vi "External Interface - Get Max & Min.vi"(0 "Ctl Refnum In":refnum<vi>, 1 "VI Refnum In":refnum<vi>, 5 "VI Name":path, 7 "String Control Value":string, 9 "Variant Control Value":variant, 11 "error in":errorcluster, 12 "Control Name":string) -> (3 "VI Refnum Out":refnum<vi>, 4 "Ctl Refnum Out":refnum<vi>, 8 "Message":string, 15 "error out":errorcluster)   [LabVIEW 2010]
panel:
  out "Type":u8
  out "Class Name":string
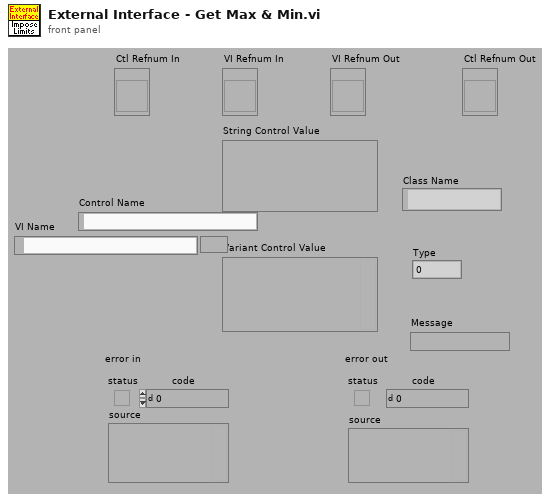
[diagram p1: front panel]
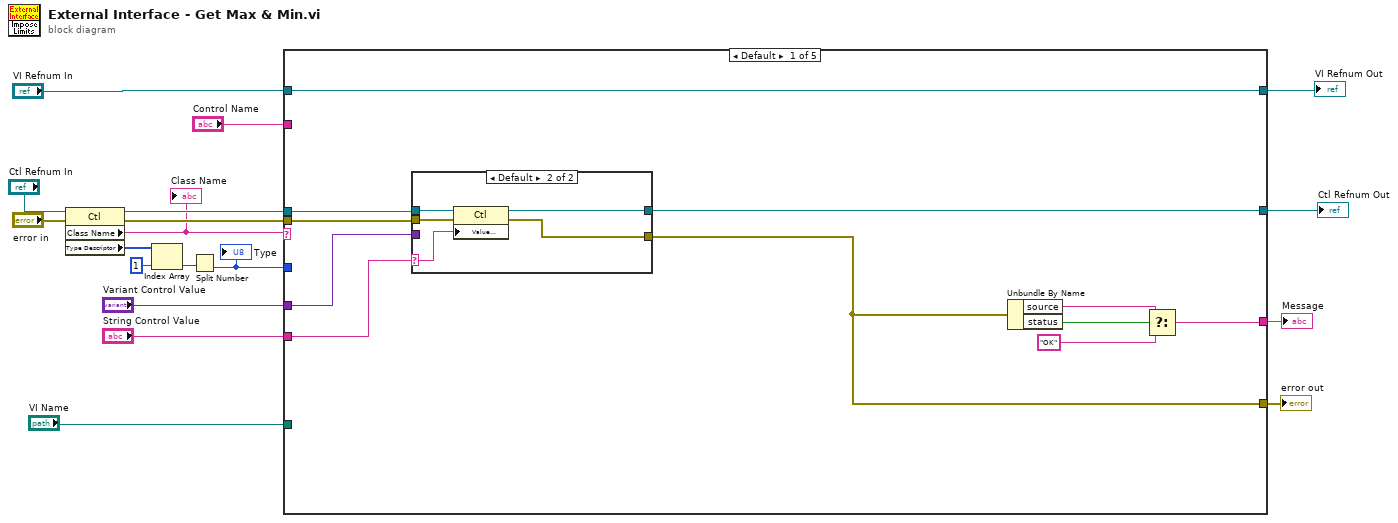
[diagram p0: block diagram]
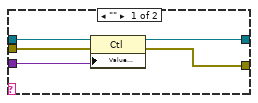
[diagram p2: hidden frame]
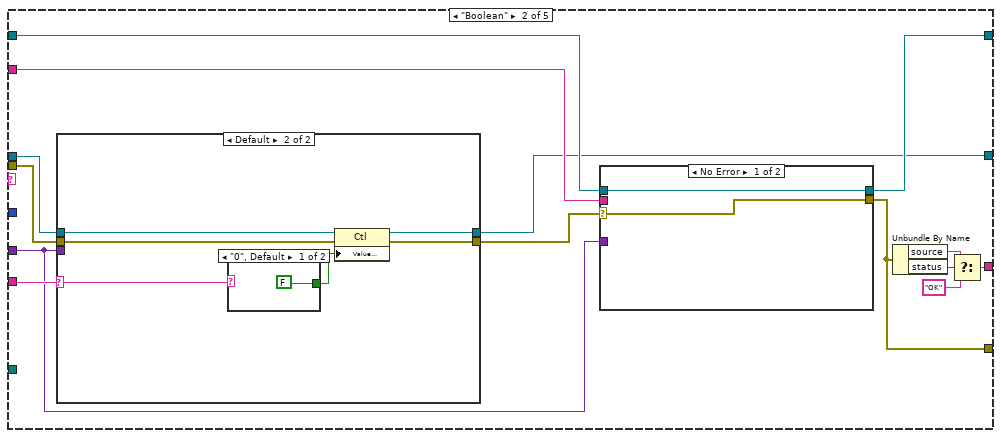
[diagram p3: hidden frame]
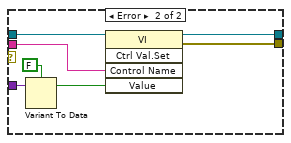
[diagram p4: hidden frame]
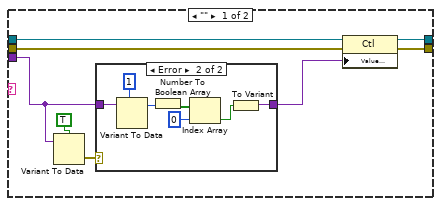
[diagram p5: hidden frame]
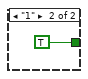
[diagram p7: hidden frame]
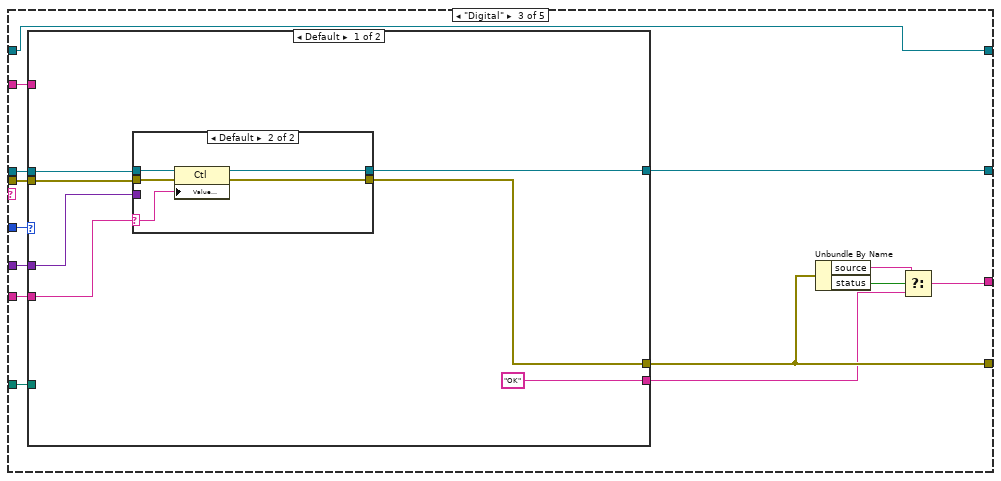
[diagram p8: hidden frame]
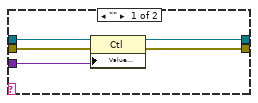
[diagram p9: hidden frame]
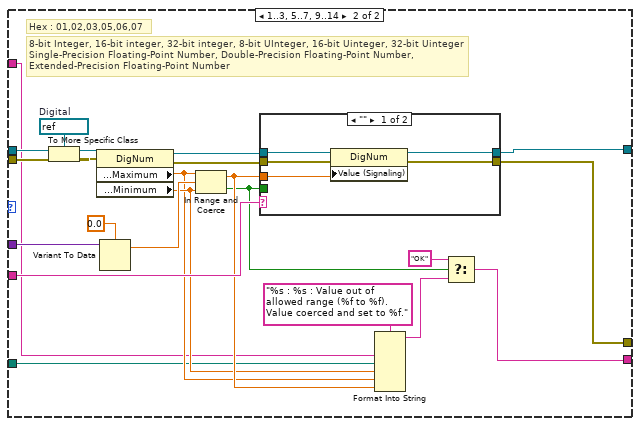
[diagram p10: hidden frame]
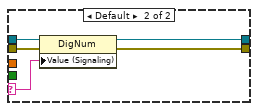
[diagram p11: hidden frame]
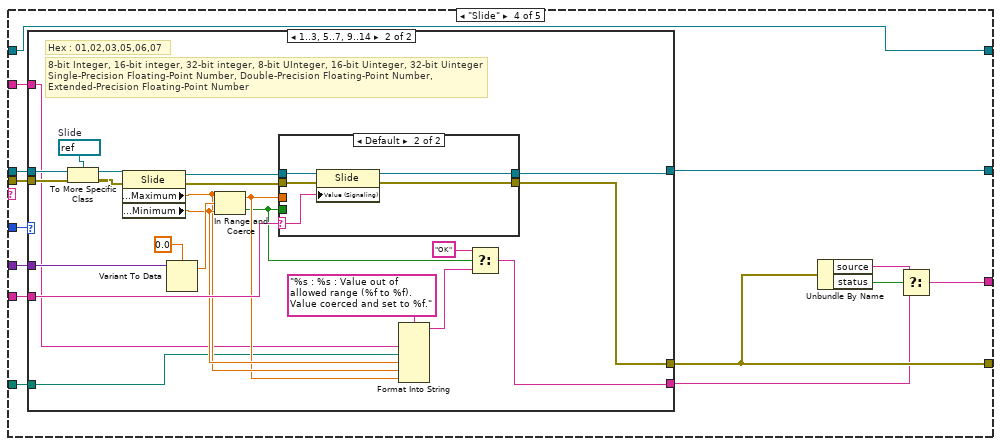
[diagram p12: hidden frame]
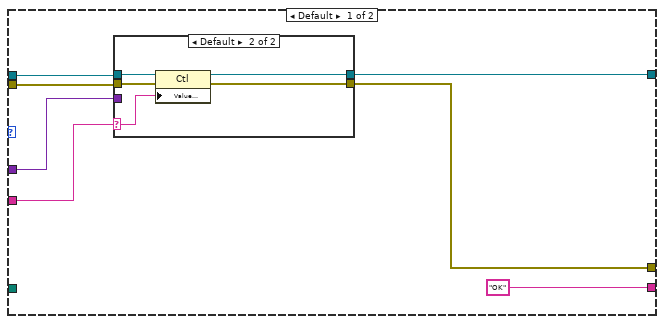
[diagram p13: hidden frame]
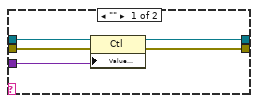
[diagram p14: hidden frame]
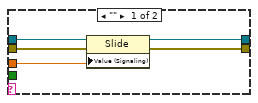
[diagram p15: hidden frame]
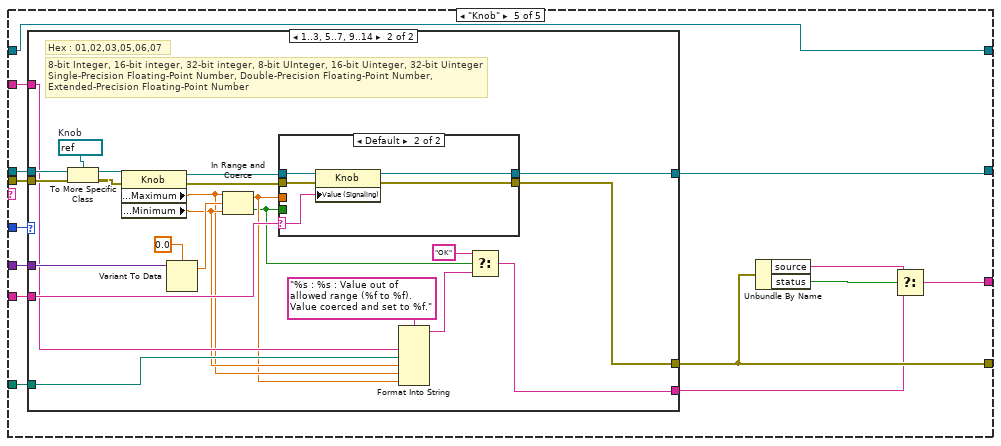
[diagram p16: hidden frame]
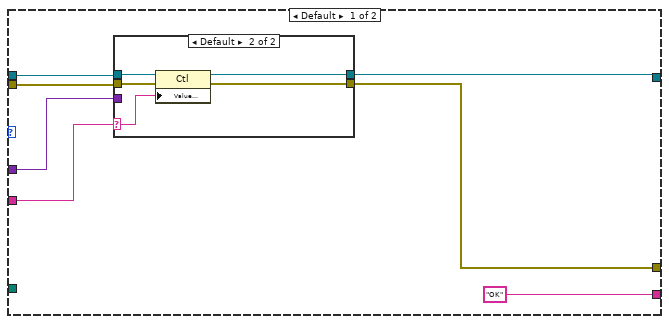
[diagram p17: hidden frame]
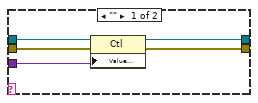
[diagram p18: hidden frame]
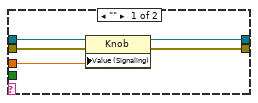
[diagram p19: hidden frame]
diagram:
  n1 = property class="Ctl"(reference="Ctl Refnum In", error in="error in") -> (reference out=w12:refnum<vi>, error out=w11:errorcluster, "Class Name"=w7:string, "Type Descriptor"=w8:i16[])
  "Class Name" <- w7
  n2 = Index Array(array=w8, index=1) -> (element=w17:i16)
  n3 = Split Number(x=w17) -> (lo(x)=w16:u8)  [unwired: 1 out]
  "Type" <- w16
  n4 = case shown="Default" w7 {
    tunnel: w16 -> [_ _ w100 w164 w228]
    tunnel: "Variant Control Value" -> [w27 w49 w99 w163 w227]
    tunnel: "String Control Value" -> [w26 w53 w98 w162 w226]
    tunnel: w12 -> [w29 w52 w97 w161 w225]
    tunnel: w11 -> [w28 w51 w96 w160 w224]
    tunnel: [w19 w44 w92 w157 w220] -> w10
    tunnel: "VI Refnum In" -> [w21 w50 w88 w152 w216]
    tunnel: "Control Name" -> [_ w48 w90 w153 w218]
    tunnel: [w24 w43 w93 w156 w221] -> w4
    tunnel: "VI Name" -> [_ _ w89 w154 w217]
    tunnel: [w21 w42 w88 w152 w216] -> w2
    tunnel: [w20 w40 w87 w151 w215] -> w1
    frame Default {
      n5 = case shown="Default" w26 {
        selector: w26 -> [_ w37]
        tunnel: w29 -> [w34 w39]
        tunnel: w28 -> [w33 w38]
        tunnel: [w31 w36] -> w19
        tunnel: w27 -> [w32 _]
        tunnel: [w30 w35] -> w20
        frame "" {
          n6 = property class="Ctl"(reference=w34, error in=w33, "Value (Signaling)"=w32) -> (reference out=w30:refnum<vi>, error out=w31:errorcluster)
        }
        frame Default {
          n7 = property class="Ctl"(reference=w39, error in=w38, "Value (Signaling)"=w37) -> (reference out=w35:refnum<vi>, error out=w36:errorcluster)
        }
      }
      n8 = Unbundle By Name(w19) -> ("source"=w22:string, "status"=w25:bool)
      n9 = Select(t=w22, s=w25, f="OK") -> (s? t:f=w24:string)
    }
    frame "Boolean" {
      n10 = case shown="Default" w53 {
        selector: w53 -> [_ w82]
        tunnel: w52 -> [w70 w84]
        tunnel: w51 -> [w69 w83]
        tunnel: [w64 w80] -> w41
        tunnel: w49 -> [w65 _]
        tunnel: [w63 w79] -> w40
        frame "" {
          n11 = Variant To Data(Variant=w65, type=TRUE) -> (error out=w68:errorcluster)  [unwired: 1 in, 1 out]
          n12 = case shown="Error" w68 {
            tunnel: w65 -> [w71 w77]
            tunnel: [w71 w73] -> w66
            frame No Error {
            }
            frame Error {
              n13 = Variant To Data(Variant=w77, type=1) -> (data=w76:i32)  [unwired: 1 in, 1 out]
              n14 = Number To Boolean Array(number=w76) -> (Boolean array=w75:bool[])
              n15 = Index Array(array=w75, index=0) -> (element=w72:bool)
              n16 = To Variant(anything=w72) -> (Variant=w73:variant)
            }
          }
          n17 = property class="Ctl"(reference=w70, error in=w69, "Value (Signaling)"=w66) -> (reference out=w63:refnum<vi>, error out=w64:errorcluster)
        }
        frame Default {
          n18 = case shown="\"0\", Default" w82 {
            tunnel: [FALSE TRUE] -> w81
            frame "0", Default {
            }
            frame "1" {
            }
          }
          n19 = property class="Ctl"(reference=w84, error in=w83, "Value (Signaling)"=w81) -> (reference out=w79:refnum<vi>, error out=w80:errorcluster)
        }
      }
      n20 = case shown="No Error" w41 {
        selector: w41 -> [w55 _]
        tunnel: w50 -> [w54 w62]
        tunnel: w49 -> [_ w60]
        tunnel: [w55 w56] -> w44
        tunnel: w48 -> [_ w61]
        tunnel: [w54 w57] -> w42
        frame No Error {
        }
        frame Error {
          n21 = Variant To Data(Variant=w60, type=FALSE) -> (data=w59:bool)  [unwired: 1 in, 1 out]
          n22 = invoke class="VI" method="Ctrl Val.Set"(reference=w62, "Control Name"=w61, "Value"=w59) -> (reference out=w57:refnum<vi>, error out=w56:errorcluster)  [unwired: 2 in, 3 out]
        }
      }
      n23 = Unbundle By Name(w44) -> ("source"=w45:string, "status"=w47:bool)
      n24 = Select(t=w45, s=w47, f="OK") -> (s? t:f=w43:string)
    }
    frame "Digital" {
      n25 = case shown="Default" w100 {
        tunnel: w97 -> [w107 w137]
        tunnel: w99 -> [w104 w134]
        tunnel: w98 -> [w105 w127]
        tunnel: w96 -> [w106 w135]
        tunnel: [w101 w118] -> w92
        tunnel: ["OK" w128] -> w91
        tunnel: w90 -> [_ w123]
        tunnel: w89 -> [_ w120]
        tunnel: [w102 w119] -> w87
        frame Default {
          n26 = case shown="Default" w105 {
            selector: w105 -> [_ w115]
            tunnel: w107 -> [w112 w117]
            tunnel: w106 -> [w111 w116]
            tunnel: [w109 w114] -> w101
            tunnel: w104 -> [w110 _]
            tunnel: [w108 w113] -> w102
            frame "" {
              n27 = property class="Ctl"(reference=w112, error in=w111, "Value (Signaling)"=w110) -> (reference out=w108:refnum<vi>, error out=w109:errorcluster)
            }
            frame Default {
              n28 = property class="Ctl"(reference=w117, error in=w116, "Value (Signaling)"=w115) -> (reference out=w113:refnum<vi>, error out=w114:errorcluster)
            }
          }
        }
        frame 1..3, 5..7, 9..14 {
          w138 = refnum<vi> refnum  # Digital
          # "8-bit Integer, 16-bit integer, 32-bit integer, 8-bit UInteger, 16-bit Uinteger, 32-bit Uinteger\nSingle-Precision Floating-Point Number, Double-Precision Floating-Point Number,\nExtended-Precision Floating-Point Number"
          # "Hex : 01,02,03,05,06,07"
          n29 = To More Specific Class(target class=w138, reference=w137, error in=w135) -> (specific class reference=w136:refnum<vi>, error out=w121:errorcluster)
          n30 = property class="DigNum"(reference=w136, error in=w121) -> (reference out=w140:refnum<vi>, error out=w139:errorcluster, "Data Entry Limits:Maximum"=w124:dbl, "Data Entry Limits:Minimum"=w125:dbl)
          n31 = Variant To Data(Variant=w134, type=0.0) -> (data=w132:dbl)  [unwired: 1 in, 1 out]
          n32 = In Range and Coerce(upper limit=w124, x=w132, lower limit=w125) -> (coerced(x)=w126:dbl, In Range?=w122:bool)
          n33 = case shown="\"\"" w127 {
            selector: w127 -> [_ w148]
            tunnel: w140 -> [w145 w150]
            tunnel: w139 -> [w144 w149]
            tunnel: [w142 w147] -> w118
            tunnel: w126 -> [w143 _]
            tunnel: w122 -> [_ _]
            tunnel: [w141 w146] -> w119
            frame "" {
              n34 = property class="DigNum"(reference=w145, error in=w144, "Value (Signaling)"=w143) -> (reference out=w141:refnum<vi>, error out=w142:errorcluster)
            }
            frame Default {
              n35 = property class="DigNum"(reference=w150, error in=w149, "Value (Signaling)"=w148) -> (reference out=w146:refnum<vi>, error out=w147:errorcluster)
            }
          }
          n36 = Format Into String(format string="%s : %s : Value out of allowed range (%f to %f). Value coerced and set to %f.", w123, w120, w125, w124, w126) -> (resulting string=w129:string)  [unwired: 2 in, 1 out]
          n37 = Select(t="OK", s=w122, f=w129) -> (s? t:f=w128:string)
        }
      }
      n38 = Unbundle By Name(w92) -> ("source"=w94:string, "status"=w95:bool)
      n39 = Select(t=w94, s=w95, f=w91) -> (s? t:f=w93:string)
    }
    frame "Slide" {
      n40 = case shown="1..3, 5..7, 9..14" w164 {
        tunnel: w161 -> [w171 w201]
        tunnel: w163 -> [w168 w197]
        tunnel: w162 -> [w169 w194]
        tunnel: w160 -> [w170 w199]
        tunnel: [w165 w182] -> w157
        tunnel: ["OK" w190] -> w155
        tunnel: w154 -> [_ w185]
        tunnel: w153 -> [_ w184]
        tunnel: [w166 w183] -> w151
        frame Default {
          n41 = case shown="Default" w169 {
            selector: w169 -> [_ w179]
            tunnel: w171 -> [w176 w181]
            tunnel: w170 -> [w175 w180]
            tunnel: [w173 w178] -> w165
            tunnel: w168 -> [w174 _]
            tunnel: [w172 w177] -> w166
            frame "" {
              n42 = property class="Ctl"(reference=w176, error in=w175, "Value (Signaling)"=w174) -> (reference out=w172:refnum<vi>, error out=w173:errorcluster)
            }
            frame Default {
              n43 = property class="Ctl"(reference=w181, error in=w180, "Value (Signaling)"=w179) -> (reference out=w177:refnum<vi>, error out=w178:errorcluster)
            }
          }
        }
        frame 1..3, 5..7, 9..14 {
          w202 = refnum<vi> refnum  # Slide
          # "8-bit Integer, 16-bit integer, 32-bit integer, 8-bit UInteger, 16-bit Uinteger, 32-bit Uinteger\nSingle-Precision Floating-Point Number, Double-Precision Floating-Point Number,\nExtended-Precision Floating-Point Number"
          # "Hex : 01,02,03,05,06,07"
          n44 = To More Specific Class(target class=w202, reference=w201, error in=w199) -> (specific class reference=w200:refnum<vi>, error out=w198:errorcluster)
          n45 = property class="Slide"(reference=w200, error in=w198) -> (reference out=w204:refnum<vi>, error out=w203:errorcluster, "Data Entry Limits:Maximum"=w188:dbl, "Data Entry Limits:Minimum"=w189:dbl)
          n46 = Variant To Data(Variant=w197, type=0.0) -> (data=w195:dbl)  [unwired: 1 in, 1 out]
          n47 = In Range and Coerce(upper limit=w188, x=w195, lower limit=w189) -> (coerced(x)=w187:dbl, In Range?=w186:bool)
          n48 = case shown="Default" w194 {
            selector: w194 -> [_ w212]
            tunnel: w204 -> [w209 w214]
            tunnel: w203 -> [w208 w213]
            tunnel: [w206 w211] -> w182
            tunnel: w187 -> [w207 _]
            tunnel: w186 -> [_ _]
            tunnel: [w205 w210] -> w183
            frame "" {
              n49 = property class="Slide"(reference=w209, error in=w208, "Value (Signaling)"=w207) -> (reference out=w205:refnum<vi>, error out=w206:errorcluster)
            }
            frame Default {
              n50 = property class="Slide"(reference=w214, error in=w213, "Value (Signaling)"=w212) -> (reference out=w210:refnum<vi>, error out=w211:errorcluster)
            }
          }
          n51 = Format Into String(format string="%s : %s : Value out of allowed range (%f to %f). Value coerced and set to %f.", w184, w185, w189, w188, w187) -> (resulting string=w191:string)  [unwired: 2 in, 1 out]
          n52 = Select(t="OK", s=w186, f=w191) -> (s? t:f=w190:string)
        }
      }
      n53 = Unbundle By Name(w157) -> ("source"=w158:string, "status"=w159:bool)
      n54 = Select(t=w158, s=w159, f=w155) -> (s? t:f=w156:string)
    }
    frame "Knob" {
      n55 = case shown="1..3, 5..7, 9..14" w228 {
        tunnel: w225 -> [w235 w265]
        tunnel: w227 -> [w232 w261]
        tunnel: w226 -> [w233 w258]
        tunnel: w224 -> [w234 w263]
        tunnel: [w229 w246] -> w220
        tunnel: ["OK" w254] -> w219
        tunnel: w218 -> [_ w253]
        tunnel: w217 -> [_ w252]
        tunnel: [w230 w247] -> w215
        frame Default {
          n56 = case shown="Default" w233 {
            selector: w233 -> [_ w243]
            tunnel: w235 -> [w240 w245]
            tunnel: w234 -> [w239 w244]
            tunnel: [w237 w242] -> w229
            tunnel: w232 -> [w238 _]
            tunnel: [w236 w241] -> w230
            frame "" {
              n57 = property class="Ctl"(reference=w240, error in=w239, "Value (Signaling)"=w238) -> (reference out=w236:refnum<vi>, error out=w237:errorcluster)
            }
            frame Default {
              n58 = property class="Ctl"(reference=w245, error in=w244, "Value (Signaling)"=w243) -> (reference out=w241:refnum<vi>, error out=w242:errorcluster)
            }
          }
        }
        frame 1..3, 5..7, 9..14 {
          w266 = refnum<vi> refnum  # Knob
          # "8-bit Integer, 16-bit integer, 32-bit integer, 8-bit UInteger, 16-bit Uinteger, 32-bit Uinteger\nSingle-Precision Floating-Point Number, Double-Precision Floating-Point Number,\nExtended-Precision Floating-Point Number"
          # "Hex : 01,02,03,05,06,07"
          n59 = To More Specific Class(target class=w266, reference=w265, error in=w263) -> (specific class reference=w264:refnum<vi>, error out=w262:errorcluster)
          n60 = property class="Knob"(reference=w264, error in=w262) -> (reference out=w268:refnum<vi>, error out=w267:errorcluster, "Data Entry Limits:Maximum"=w250:dbl, "Data Entry Limits:Minimum"=w251:dbl)
          n61 = Variant To Data(Variant=w261, type=0.0) -> (data=w259:dbl)  [unwired: 1 in, 1 out]
          n62 = In Range and Coerce(upper limit=w250, x=w259, lower limit=w251) -> (coerced(x)=w249:dbl, In Range?=w248:bool)
          n63 = case shown="Default" w258 {
            selector: w258 -> [_ w276]
            tunnel: w268 -> [w273 w278]
            tunnel: w267 -> [w272 w277]
            tunnel: [w270 w275] -> w246
            tunnel: w249 -> [w271 _]
            tunnel: w248 -> [_ _]
            tunnel: [w269 w274] -> w247
            frame "" {
              n64 = property class="Knob"(reference=w273, error in=w272, "Value (Signaling)"=w271) -> (reference out=w269:refnum<vi>, error out=w270:errorcluster)
            }
            frame Default {
              n65 = property class="Knob"(reference=w278, error in=w277, "Value (Signaling)"=w276) -> (reference out=w274:refnum<vi>, error out=w275:errorcluster)
            }
          }
          n66 = Format Into String(format string="%s : %s : Value out of allowed range (%f to %f). Value coerced and set to %f.", w253, w252, w251, w250, w249) -> (resulting string=w255:string)  [unwired: 2 in, 1 out]
          n67 = Select(t="OK", s=w248, f=w255) -> (s? t:f=w254:string)
        }
      }
      n68 = Unbundle By Name(w220) -> ("source"=w222:string, "status"=w223:bool)
      n69 = Select(t=w222, s=w223, f=w219) -> (s? t:f=w221:string)
    }
  }
  "error out" <- w10
  "Ctl Refnum Out" <- w1
  "VI Refnum Out" <- w2
  "Message" <- w4
